vi "Calc T0.vi"(6 "Setting":T1={"P [MPa]"=0.0, "A [MPa/V]"=0.0, "P0 [MPa]"=0.0, "P start [%]"=4.0, "P end [%]"=3.5, "T0 DUT [s]"=0.0, "T0 CMBR [s]"=0.0} {"P0 [MPa]" format="%#_13g"; "A [MPa/V]" format="%#_13g"}, 7 "init":bool, 11 "P":dbl) -> (0 "done":bool, 3 "T0":dbl format="%0.2f")   [LabVIEW 2019]
uses:
  TypeDef/Setting Pressure PI.ctl
  <vilib>/ptbypt/NI_PtbyPt.lvlib
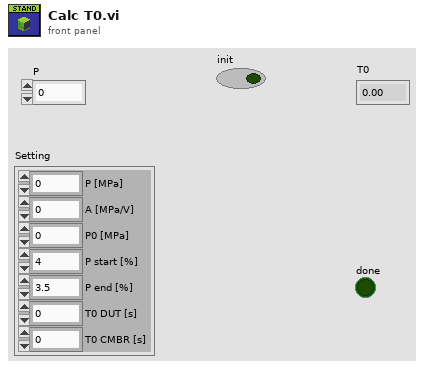
[diagram p1: front panel]
types:
  T1 = typedef "Setting Pressure PI.ctl" = cluster{"P [MPa]":dbl, "A [MPa/V]":dbl, "P0 [MPa]":dbl, "P start [%]":dbl, "P end [%]":dbl, "T0 DUT [s]":dbl, "T0 CMBR [s]":dbl}
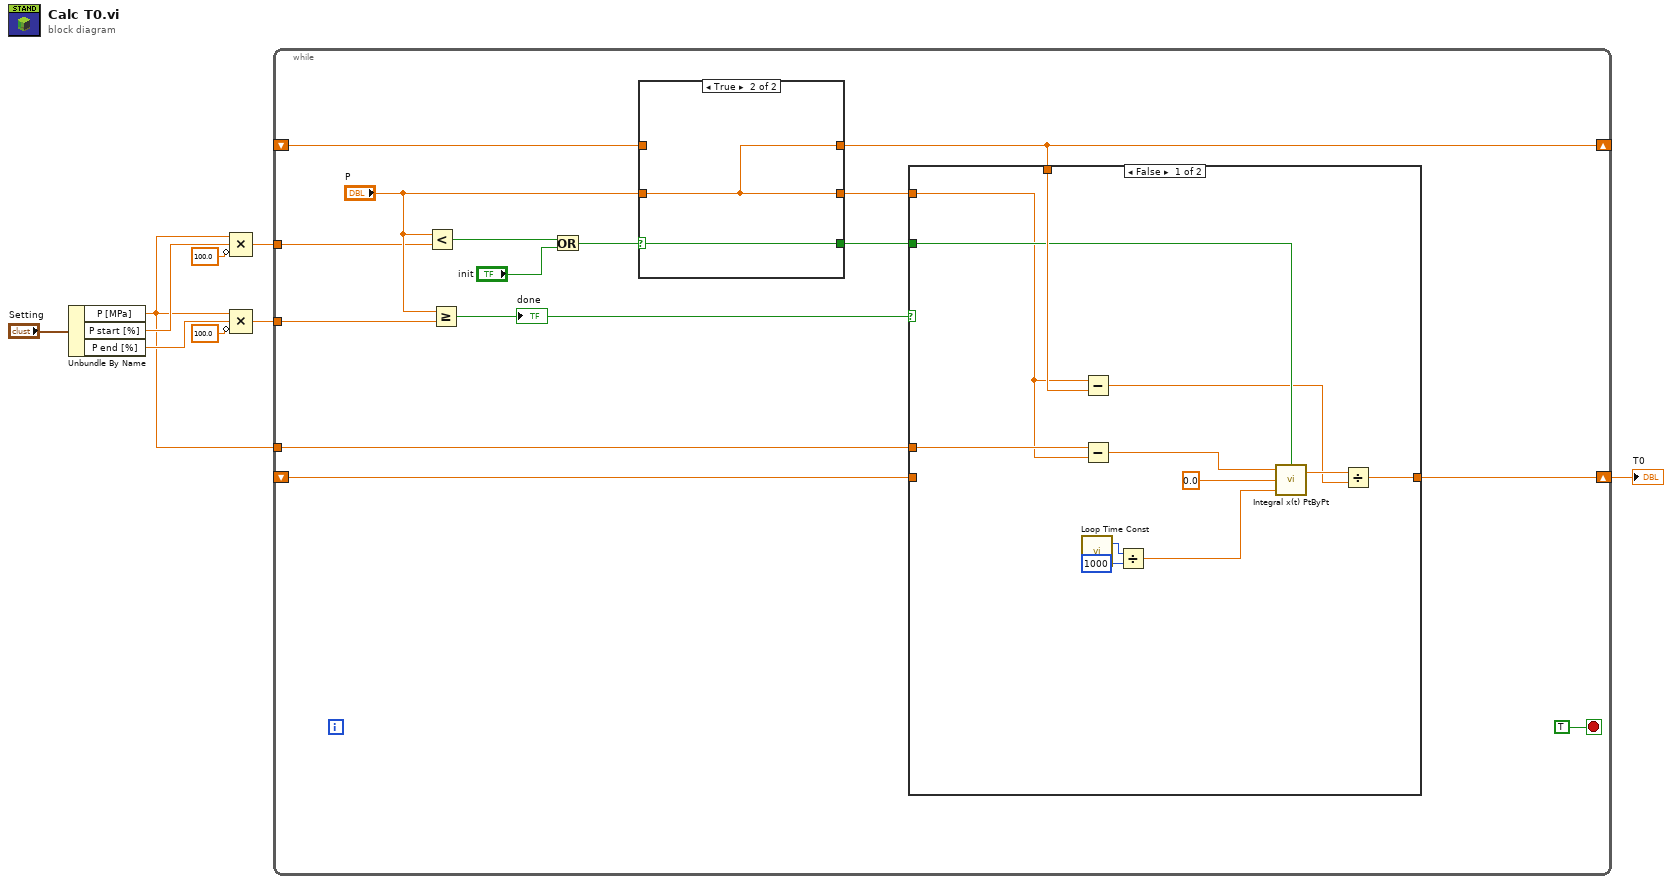
[diagram p0: block diagram]
diagram:
  n1 = Unbundle By Name("Setting") -> ("P [MPa]"=w1:dbl, "P start [%]"=w7:dbl, "P end [%]"=w3:dbl)
  n2 = Compound Arithmetic op=MULTIPLY(w1, w7, invert 100.0 ("value")) -> (w6:dbl)
  n3 = Compound Arithmetic op=MULTIPLY(w1, w3, invert 100.0 ("value")) -> (w2:dbl)
  n4 = while {
    shift-right: [w12] -> _
    shift-left: _ -> [w21]
    tunnel: w6 -> [w18]
    tunnel: w2 -> [w17]
    shift-right: [w16] -> w9
    shift-left: _ -> [w13]
    tunnel: w1 -> [w10]
    stop <- TRUE stop-if-true
    n5 = Less?(x="P", y=w18) -> (x < y?=w23:bool)
    n6 = Greater Or Equal?(x="P", y=w17) -> (x >= y?=w15:bool)
    "done" <- w15
    n7 = Or(x=w23, y="init") -> (x .or. y?=w20:bool)
    n8 = case shown="True" w20 {
      selector: w20 -> [w38 w41]
      tunnel: "P" -> [w40 w42]
      tunnel: [w40 w42] -> w14
      tunnel: [w39 w42] -> w12
      tunnel: w21 -> [w39 _]
      tunnel: [w38 w41] -> w11
      frame False {
      }
      frame True {
      }
    }
    n9 = case shown="False" w15 {
      tunnel: [w26 w37] -> w16
      tunnel: w14 -> [w27 _]
      tunnel: w13 -> [_ w37]
      tunnel: w12 -> [w31 _]
      tunnel: w11 -> [w30 _]
      tunnel: w10 -> [w29 _]
      frame False {
        n10 = call "Loop Time Const.vi"() -> ("loop time ms"=w36:i64)  [unwired: 3 in]
        n11 = Subtract(x=w27, y=w31) -> (x-y=w25:dbl)
        n12 = Subtract(x=w29, y=w27) -> (x-y=w28:dbl)
        n13 = Divide(x=w36, y=i64 1000) -> (x/y=w35:dbl)
        n14 = call <vilib>:"Integral x(t) PtByPt.vi"("initialize"=w30, "dt"=w35, "initial condition"=0.0, "x"=w28) -> ("integral x(t)"=w32:dbl)  [unwired: 1 out]
        n15 = Divide(x=w32, y=w25) -> (x/y=w26:dbl)
      }
      frame True {
      }
    }
  }
  "T0" <- w9
